vi "CheckAlarmAcquisitionSettings.vi"(8 "error in (no error)":errorcluster, 9 "acq config in":T1, 10 "collection reason":string, 11 "map":T5) -> (0 "error out":errorcluster, 1 "acq config out":T1)   [LabVIEW 2017, in "McsaDataEventCreator.lvlib"]
uses:
  <vilib>/addons/InsightCM/Devices/Shared/Mcsa/McsaDataEventCreator/McsaDataEventCreator.lvlib
  <vilib>/addons/PointValueMap/controls/PointMap.ctl
  <vilib>/addons/InsightCM/Devices/Shared/Mcsa/McsaDataEventCreator/controls/AcqParams.ctl
  <vilib>/addons/InsightCM/Devices/Shared/Common/DataAccumulator/controls/AccumulationSettings.ctl
  <vilib>/addons/InsightCM/Devices/Shared/Common/DataAccumulator/controls/accumulationType.ctl
  <vilib>/addons/InsightCM/Devices/Shared/Common/DVRBuffer/controls/BufferLocation.ctl
  <vilib>/addons/InsightCM/Devices/Shared/Common/DataEventCreator/controls/Reason.ctl
  <vilib>/addons/PointValueMap/subVIs/Point_Read_i32.vi
  <vilib>/addons/InsightCM/Devices/Shared/Common/DataEventCreator/DataEventCreator.lvlib
  <vilib>/addons/PointValueMap/PointValueMap.lvlib
  <vilib>/addons/InsightCM/Devices/Shared/Common/DataAccumulator/DataAccumulator.lvlib
  <vilib>/addons/InsightCM/Devices/Shared/Common/DVRBuffer/DVRBuffer.lvlib
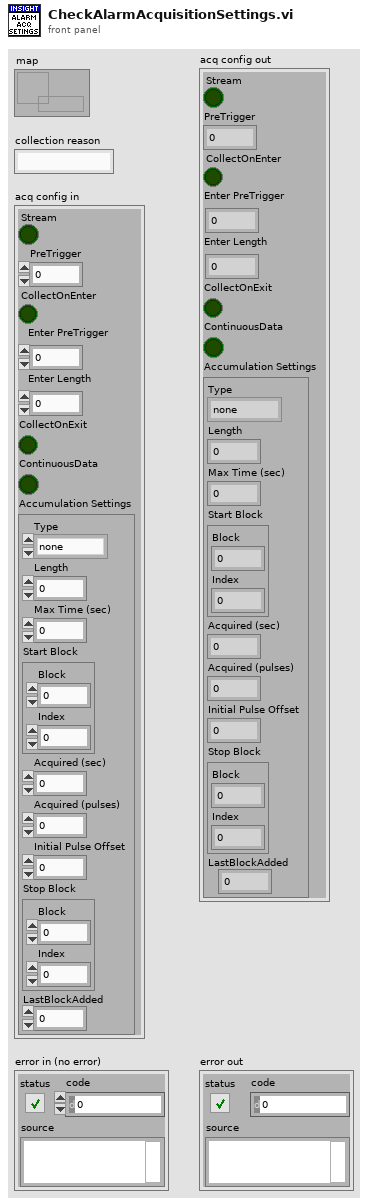
[diagram p1: front panel]
types:
  T1 = typedef "McsaDataEventCreator.lvlib/AcqParams.ctl" = cluster{"Stream":bool, "PreTrigger":i32, "CollectOnEnter":bool, "Enter PreTrigger":i32, "Enter Length":dbl, "CollectOnExit":bool, "ContinuousData":bool, "Accumulation Settings":T2}
  T2 = typedef "DataAccumulator.lvlib/AccumulationSettings.ctl" = cluster{"Type":T3, "Length":dbl, "Max Time (sec)":dbl, "Start Block":T4, "Acquired (sec)":dbl, "Acquired (pulses)":i32, "Initial Pulse Offset":dbl, "Stop Block":T4, "LastBlockAdded":u32}
  T3 = typedef "DataAccumulator.lvlib/accumulationType.ctl" = enum16{"none", "seconds", "revolutions"}
  T4 = typedef "DVRBuffer.lvlib/BufferLocation.ctl" = cluster{"Block":u32, "Index":i32}
  T5 = typedef "PointValueMap.lvlib/PointMap.ctl" = refnum<data-value>
  T6 = typedef "DataEventCreator.lvlib/Reason.ctl" = enum16{"Periodic Event", "Delta EU Event", "Trend Event", "Alarm Event", "User Event", "Enter Operating State", "Exit Operating State", "Multiple Events", "Other"}
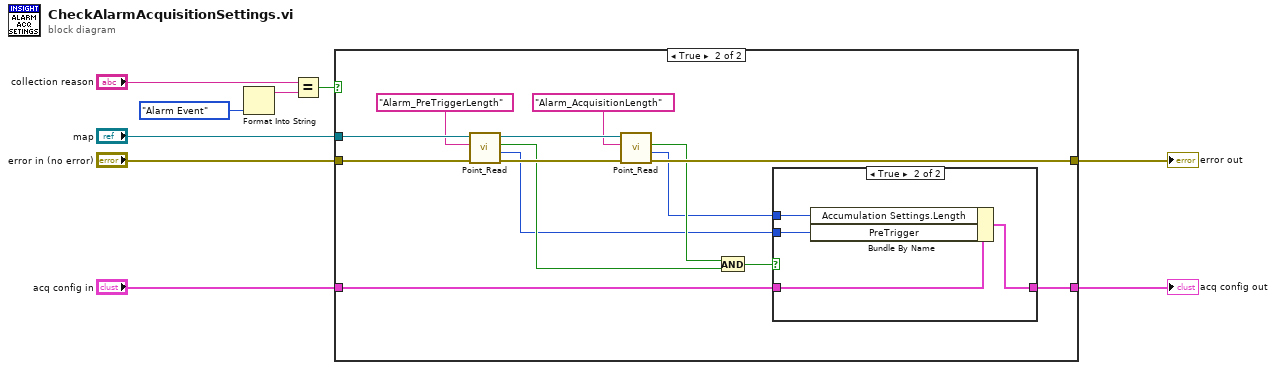
[diagram p0: block diagram]
diagram:
  n1 = Format Into String(Reason."Alarm Event" ("Reason")) -> (resulting string=w7:string)  [unwired: 3 in, 1 out]
  n2 = Equal?(x="collection reason", y=w7) -> (x = y?=w6:bool)
  n3 = case shown="True" w6 {
    tunnel: "map" -> [_ w25]
    tunnel: "error in (no error)" -> [w11 w24]
    tunnel: [w11 w21] -> w3
    tunnel: "acq config in" -> [w10 w15]
    tunnel: [w10 w12] -> w1
    frame False {
    }
    frame True {
      n4 = call-poly <vilib>:"Point_Read.vi"("Error In"=w24, "Tag"="Alarm_PreTriggerLength", "Map"=w25) -> ("Error Out"=w22:errorcluster, "Value"=w13:i32, "Found?"=w17:bool, "Map Out"=w23:T5)  [unwired: 3 in, 2 out]
      n5 = call-poly <vilib>:"Point_Read.vi"("Error In"=w22, "Tag"="Alarm_AcquisitionLength", "Map"=w23) -> ("Error Out"=w21:errorcluster, "Value"=w14:i32, "Found?"=w18:bool)  [unwired: 3 in, 3 out]
      n6 = And(x=w18, y=w17) -> (x .and. y?=w16:bool)
      n7 = case shown="True" w16 {
        tunnel: w15 -> [w26 w30]
        tunnel: w14 -> [_ w28]
        tunnel: w13 -> [_ w27]
        tunnel: [w26 w29] -> w12
        frame False {
        }
        frame True {
          n8 = Bundle By Name(cluster=w30, "Accumulation Settings.Length"=w28, "PreTrigger"=w27) -> (w29:T1)
        }
      }
    }
  }
  "acq config out" <- w1
  "error out" <- w3
